vi "FMV - get control details.vi"(8 "error in (no error)":errorcluster) -> (0 "error out":errorcluster, 3 "Control details":string)   [LabVIEW 2020, in "ui-testing.lvlib"]
uses:
  ui-testing.lvlib
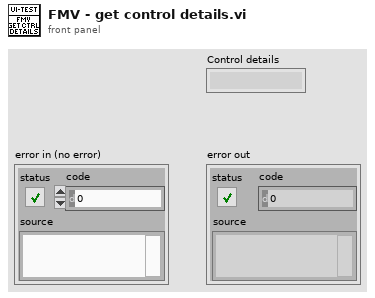
[diagram p1: front panel]
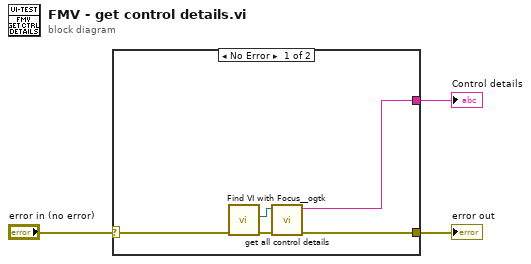
[diagram p0: block diagram]
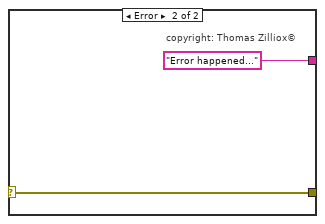
[diagram p2: hidden frame]
diagram:
  n1 = case shown="No Error" "error in (no error)" {
    selector: "error in (no error)" -> [w8 w10]
    tunnel: [w5 w10] -> w2
    tunnel: [w4 "Error happened..."] -> w1
    frame No Error {
      n2 = call <userlib>:"Find VI with Focus__ogtk.vi"("error in"=w8) -> ("error out"=w6:errorcluster, "VI with Focus"=w7:refnum<vi>)  [unwired: 6 in, 3 out]
      n3 = call "get all control details.vi"("error in"=w6, "VI (Caller)"=w7) -> ("error out"=w5:errorcluster, "Control details"=w4:string)  [unwired: 8 in]
    }
    frame Error {
      # "copyright: Thomas Zilliox©"
    }
  }
  "error out" <- w2
  "Control details" <- w1
